vi "get production information.vi"() -> (0 "fail":i32, 1 "pass":i32, 3 "type":string)   [LabVIEW 2014]
uses:
  <vilib>/Utility/file.llb/Read From Spreadsheet File (string).vi
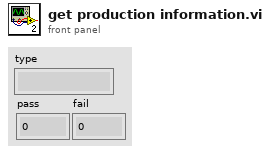
[diagram p1: front panel]
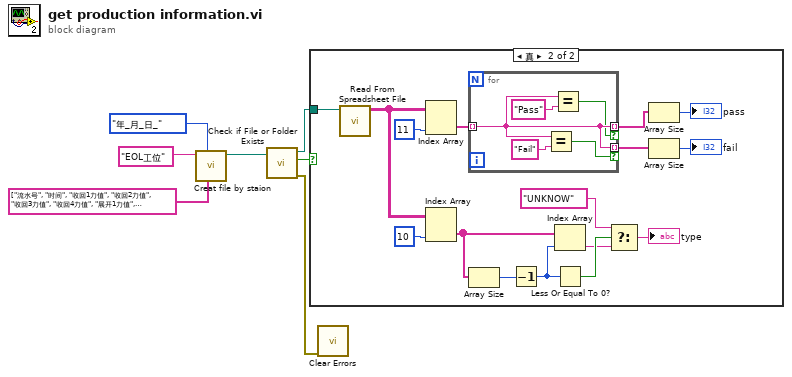
[diagram p0: block diagram]
diagram:
  n1 = call "Creat file by staion.vi"("Header"=string[] ["流水号", "时间", "收回1力值", "收回2力值", "收回3力值", "收回4力值", "展开1力值", "展开2力值", "展开3力值", "展开4力值", "项目号", "Pass/Fail"], "basis as"=enum16{"年_", "年_月_日_"}."年_月_日_", "station"="EOL工位" ("file name")) -> ("new file path (Not A Path if cancelled)"=w5:path)  [unwired: 8 in]
  n2 = call <vilib>:"Check if File or Folder Exists.vi"("path"=w5) -> ("error out"=w1:errorcluster, "file or folder exists?"=w7:bool, "dup path"=w6:path)  [unwired: 8 in]
  n3 = case shown="真" w7 {
    tunnel: w6 -> [_ w8]
    frame False {
    }
    frame True {
      n4 = call-poly <vilib>:"Read From Spreadsheet File.vi"("file path (dialog if empty)"=w8) -> ("all rows"=w15:string[][])  [unwired: 6 in, 4 out]
      n5 = Index Array(array=w15, index (col)=11 ("禁用的索引 (列)")) -> (element=w13:string[])  [unwired: 1 in]
      n6 = Index Array(array=w15, index (col)=10 ("禁用的索引 (列)")) -> (element=w19:string[])  [unwired: 1 in]
      n7 = for {
        tunnel: w13 -> [w25] mode=indexing
        tunnel: [w25] -> w12 mode=indexing if=w26
        tunnel: [w25] -> w11 mode=indexing if=w24
        n8 = Equal?(x=w25, y="Fail") -> (x = y?=w26:bool)
        n9 = Equal?(x=w25, y="Pass") -> (x = y?=w24:bool)
      }
      n10 = Array Size(array=w19) -> (size(s)=w20:i32)
      n11 = Decrement(x=w20) -> (x-1=w22:i32)
      n12 = Index Array(array=w19, index=w22) -> (element=w21:string)
      n13 = Less Or Equal To 0?(x=w22) -> (x <= 0?=w23:bool)
      n14 = Select(t="UNKNOW", s=w23, f=w21) -> (s? t:f=→"type":string)
      n15 = Array Size(array=w11) -> (size(s)=→"pass":i32)
      n16 = Array Size(array=w12) -> (size(s)=→"fail":i32)
    }
  }
  n17 = call <vilib>:"Clear Errors.vi"("error in (no error)"=w1) -> ()  [unwired: 5 in, 2 out]
